vi "Dual_DM_Control_Main_V5.vi"() -> ()   [LabVIEW 2014]
uses:
  Controls/MirrorModes.ctl
  Controls/Standard Action.ctl
  <vilib>/Analysis/baseanly.llb/Mean (DBL).vi
  <vilib>/Utility/file.llb/Write To Spreadsheet File (DBL).vi
  <vilib>/Utility/file.llb/Read From Spreadsheet File (DBL).vi
  <vilib>/Analysis/NI_AALBase.lvlib
panel:
  in  "Control Mode":T1(radio)
  in  "Active Mirror":enum32{"Mirror 1", "Mirror 2"}(radio)
  in  "Clear Modes":bool
  in  "Mirror Modes":T2
  in  "Load Modes":bool
  in  "Save Modes":bool
  in  "Scan Modes":bool
  in  "Load Flat":bool
  in  "Apply Zero":bool
  in  "Load V Map":bool
  in  "Save V Map":bool
  in  "Apply Flat":bool
  in  "Center Bias":bool
  in  "Exit":bool
  out "Pixel Map (-1 to 1)":dbl[][](graph)
  # "Mode"
  # "Amount (nm)"
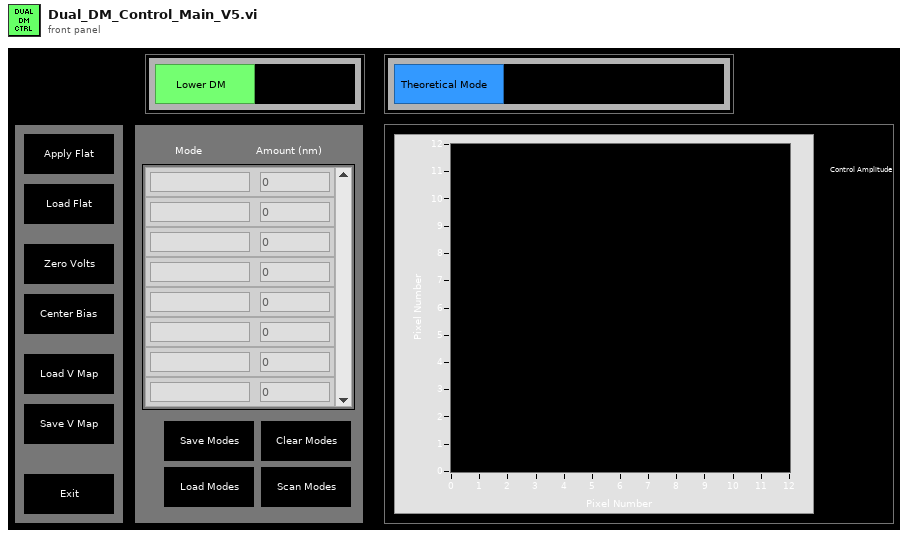
[diagram p1: front panel]
types:
  T1 = enum32{"Theoretical Mode", "Practical Mode", "Poke"}
  T2 = typedef "MirrorModes.ctl" = cluster{"Mode":string, "Amplitude":dbl}[]
  T3 = typedef "Standard Action.ctl" = enum16{"Read", "Write"}
  T4 = typedef "MirrorModes_DUAL.ctl" = cluster{"Mode":string, "Amplitude":dbl}[][]
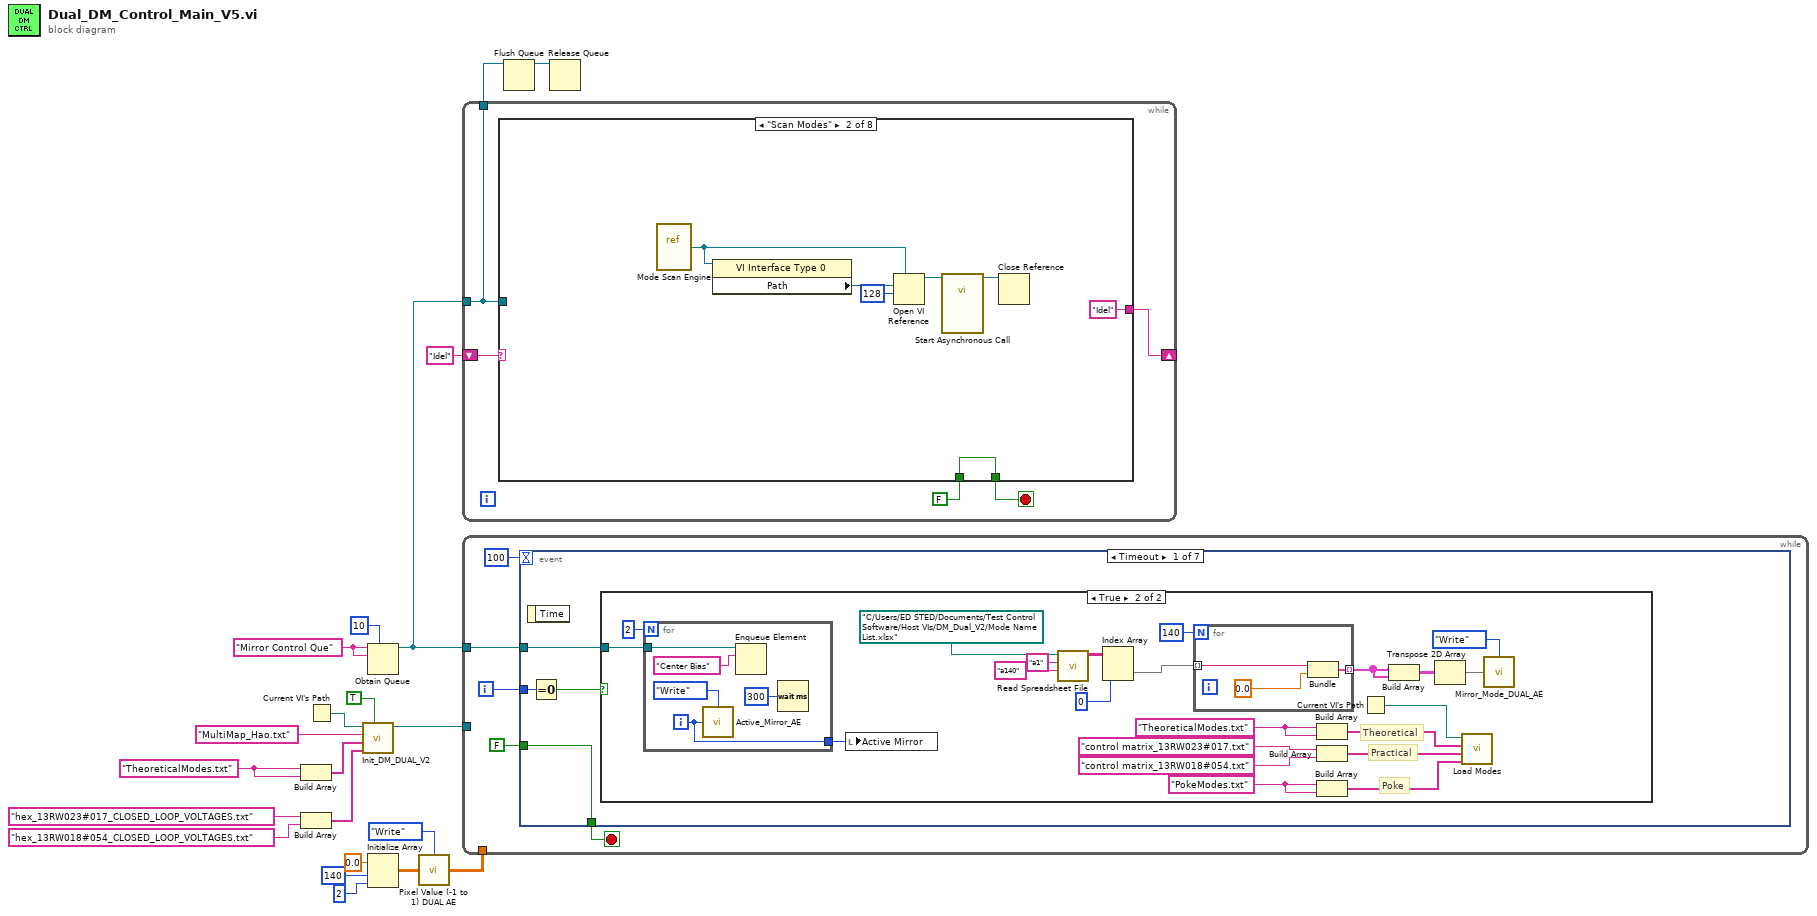
[diagram p0: block diagram]
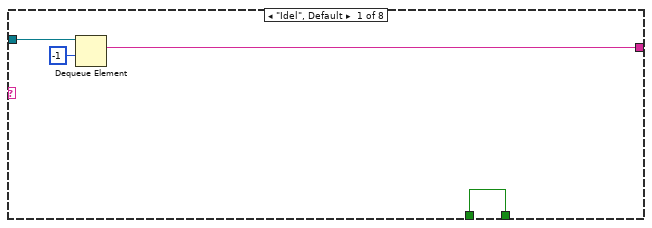
[diagram p2: hidden frame]
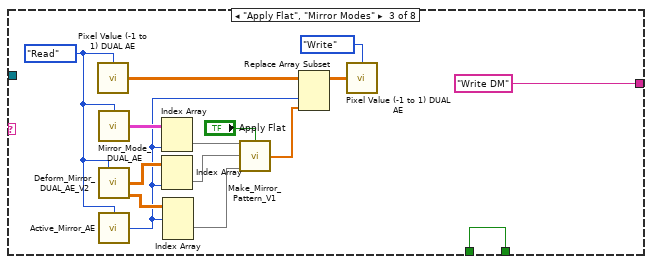
[diagram p3: hidden frame]
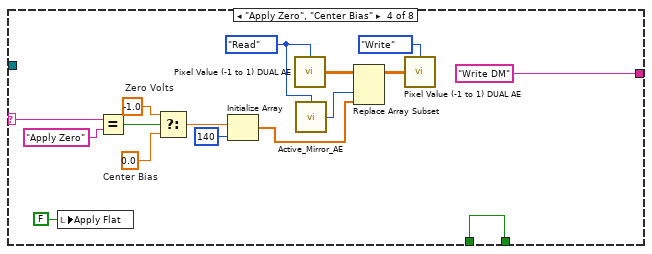
[diagram p4: hidden frame]
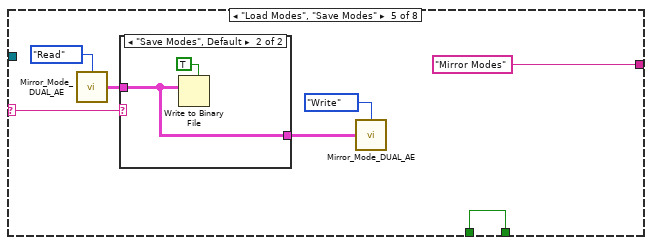
[diagram p5: hidden frame]
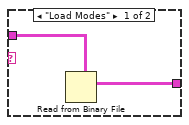
[diagram p6: hidden frame]
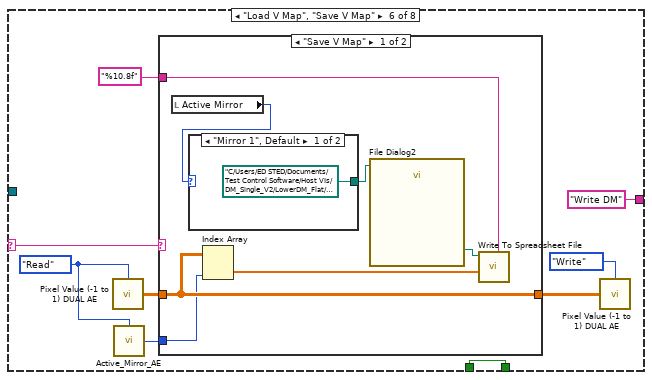
[diagram p7: hidden frame]
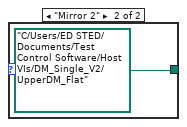
[diagram p8: hidden frame]
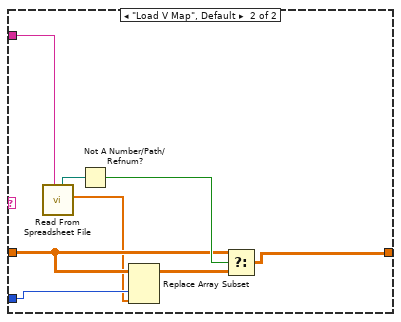
[diagram p9: hidden frame]
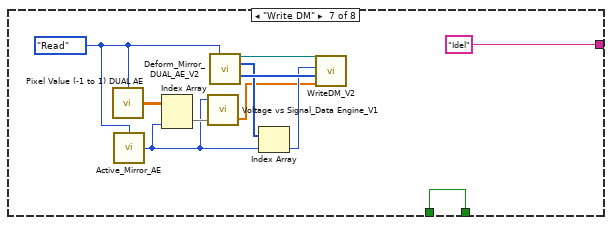
[diagram p10: hidden frame]
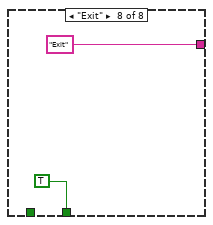
[diagram p11: hidden frame]
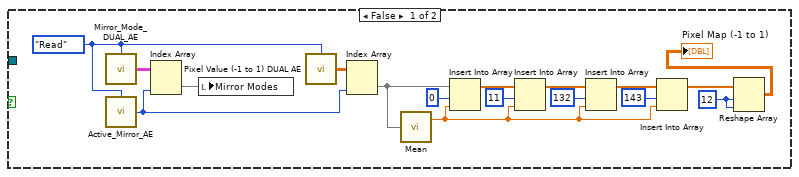
[diagram p12: hidden frame]
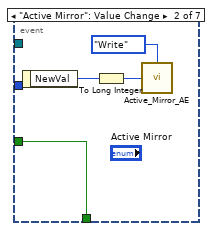
[diagram p13: hidden frame]
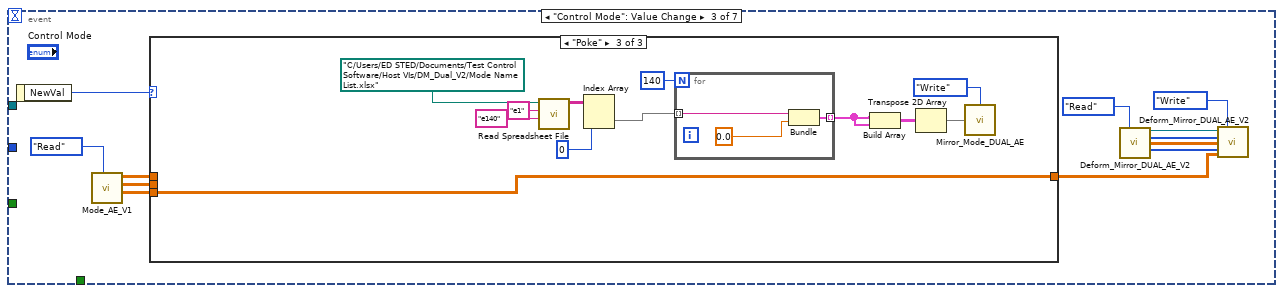
[diagram p14: hidden frame]
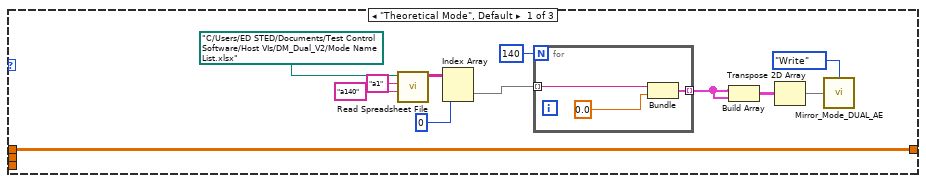
[diagram p15: hidden frame]
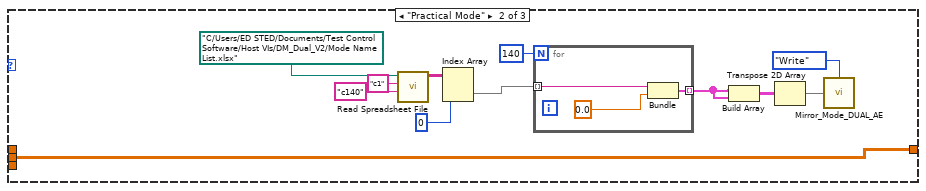
[diagram p16: hidden frame]
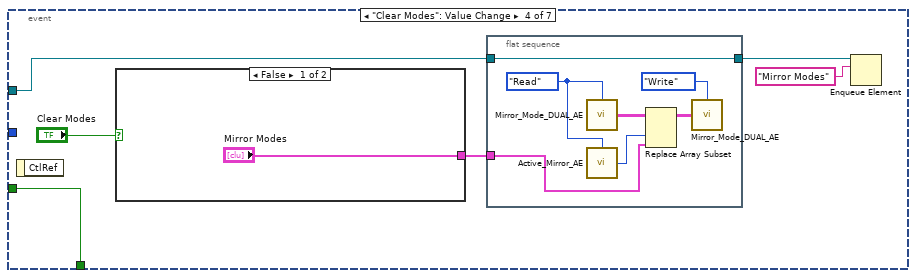
[diagram p17: hidden frame]
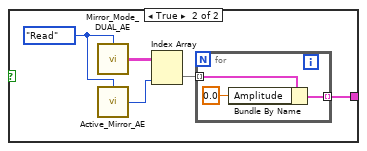
[diagram p18: hidden frame]
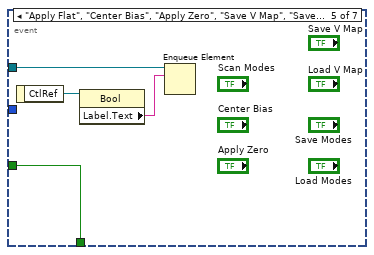
[diagram p19: hidden frame]
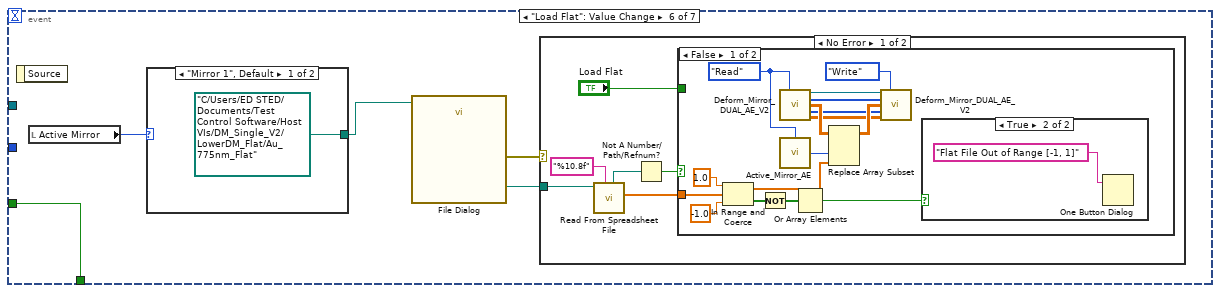
[diagram p20: hidden frame]
diagram:
  w1 = "TheoreticalModes.txt" ("name or relative path")
  w21 = "Mirror Control Que" ("name (unnamed)")
  n1 = Build Array(w1, w1) -> (w2:string[])
  n2 = Build Array("hex_13RW023#017_CLOSED_LOOP_VOLTAGES.txt" ("name or relative path"), "hex_13RW018#054_CLOSED_LOOP_VOLTAGES.txt" ("name or relative path")) -> (w11:string[])
  n3 = Current VI's Path() -> (path=w13:path)
  n4 = call "Init_DM_DUAL_V2.vi"("BM Flat"=TRUE, "BM Flat File"=w11, "Control Mode In"=w2, "DM Mapping File"="MultiMap_Hao.txt" ("name or relative path"), "Base File Path"=w13) -> ("reference out"=w19:refnum<k7>)  [unwired: 6 in]
  n5 = Obtain Queue(max queue size (-1, unlimited)=10, name (unnamed)=w21, element data type=w21) -> (queue out=w15:refnum<queue>)  [unwired: 2 in, 2 out]
  n6 = Initialize Array(0.0 ("element"), 140 ("dimension size"), 2 ("dimension size")) -> (w7:dbl[][])
  n7 = call "Pixel Value (-1 to 1) DUAL AE.vi"("Action"=Standard_Action."Write", "Pixel Value (-1 to 1)"=w7) -> ("Pixel Value (-1 to 1) Out"=w5:dbl[][])  [unwired: 13 in]
  n8 = while {
    tunnel: w15 -> [w22]
    shift-right: [w26] -> _
    shift-left: "Idel" ("name (unnamed)") -> [w25]
    tunnel: [w22] -> w18
    stop <- w24 stop-if-true
    n9 = case shown="\"Scan Modes\"" w25 {
      selector: w25 -> [_ _ _ w64 w71 w87 _ _]
      tunnel: w22 -> [w30 _ _ _ _ _ _ _]
      tunnel: [w28 "Idel" ("name (unnamed)") "Write DM" ("name (unnamed)") "Write DM" ("name (unnamed)") "Mirror Modes" ("name (unnamed)") "Write DM" ("name (unnamed)") "Idel" ("name (unnamed)") "Exit" ("name (unnamed)")] -> w26
      tunnel: [w27 w36 w51 w68 w75 w88 w116 TRUE] -> w24
      tunnel: FALSE -> [w27 w36 w51 w68 w75 w88 w116 _]
      frame "Idel", Default {
        n10 = Dequeue Element(queue=w30, timeout in ms (-1)=-1) -> (element=w28:string)  [unwired: 1 in, 3 out]
      }
      frame "Scan Modes" {
        n11 = vi-ref "Mode Scan Engine.vi"() -> (w31:refnum<vi>)
        n12 = property class="VI Interface Type 0"(reference=w31) -> ("Path"=w32:path)  [unwired: 1 in, 2 out]
        n13 = Open VI Reference(type specifier VI Refnum (for type only)=w31, vi path=w32, options=128) -> (vi reference=w34:refnum<vi>)  [unwired: 3 in, 1 out]
        n14 = call-by-ref "Start Asynchronous Call"(reference=w34) -> (reference out=w35:refnum<vi>)  [unwired: 3 in, 1 out]
        n15 = Close Reference(reference=w35) -> ()  [unwired: 1 in, 1 out]
      }
      frame "Apply Flat", "Mirror Modes" {
        w47 = Standard_Action."Read" ("Action")
        n16 = call "Pixel Value (-1 to 1) DUAL AE.vi"("Action"=w47) -> ("Pixel Value (-1 to 1) Out"=w48:dbl[][])  [unwired: 14 in]
        n17 = call "Mirror_Mode_DUAL_AE.vi"("Action"=w47) -> ("Mirror Modes Out"=w44:T4)  [unwired: 14 in]
        n18 = call "Deform_Mirror_DUAL_AE_V2.vi"("Action"=w47) -> ("Flat Files Out"=w42:dbl[][], "Mode Matrix Out"=w40:dbl[][][])  [unwired: 10 in, 3 out]
        n19 = call "Active_Mirror_AE.vi"("Action"=w47) -> ("Active Mirror"=w38:i32)  [unwired: 14 in]
        n20 = Index Array(array=w44, index (col)=w38) -> (element=w45:cluster{"Mode":string, "Amplitude":dbl}[])  [unwired: 1 in]
        n21 = Index Array(array=w42, index (col)=w38) -> (element=w43:dbl[])  [unwired: 1 in]
        n22 = Index Array(array=w40, index (dim 0)=w38) -> (element=w39:dbl[][])  [unwired: 2 in]
        n23 = call "Make_Mirror_Pattern_V1.vi"("Mirror Modes In"=w45, "Flat On?"="Apply Flat", "Flat File In"=w43, "Mirror Modes Array"=w39) -> ("Pixel Value U (-1 to 1)"=w49:dbl[])  [unwired: 11 in]
        n24 = Replace Array Subset(array=w48, new element=w49, index (col)=w38) -> (w50:dbl[][])  [unwired: 1 in]
        n25 = call "Pixel Value (-1 to 1) DUAL AE.vi"("Action"=Standard_Action."Write", "Pixel Value (-1 to 1)"=w50) -> ()  [unwired: 13 in, 1 out]
      }
      frame "Apply Zero", "Center Bias" {
        w57 = Standard_Action."Read" ("Action")
        w60 = -1.0  # Zero Volts
        w62 = 0.0  # Center Bias
        n26 = local write "Apply Flat"(FALSE ("Apply Flat")) -> ()
        n27 = Equal?(x=w64, y="Apply Zero") -> (x = y?=w63:bool)
        n28 = Select(t=w60, s=w63, f=w62) -> (s? t:f=w61:dbl)
        n29 = Initialize Array(w61, 140 ("dimension size")) -> (w54:dbl[])
        n30 = call "Pixel Value (-1 to 1) DUAL AE.vi"("Action"=w57) -> ("Pixel Value (-1 to 1) Out"=w55:dbl[][])  [unwired: 14 in]
        n31 = call "Active_Mirror_AE.vi"("Action"=w57) -> ("Active Mirror"=w56:i32)  [unwired: 14 in]
        n32 = Replace Array Subset(array=w55, new element=w54, index (col)=w56) -> (w58:dbl[][])  [unwired: 1 in]
        n33 = call "Pixel Value (-1 to 1) DUAL AE.vi"("Action"=Standard_Action."Write", "Pixel Value (-1 to 1)"=w58) -> ()  [unwired: 13 in, 1 out]
      }
      frame "Load Modes", "Save Modes" {
        n34 = call "Mirror_Mode_DUAL_AE.vi"("Action"=Standard_Action."Read") -> ("Mirror Modes Out"=w70:T4)  [unwired: 14 in]
        n35 = case shown="\"Save Modes\", Default" w71 {
          tunnel: w70 -> [w77 w78]
          tunnel: [w76 w78] -> w69
          frame "Load Modes" {
            n36 = Read from Binary File(5:w77) -> (2:w76:T4)  [unwired: 5 in, 3 out]
          }
          frame "Save Modes", Default {
            n37 = Write to Binary File(data=w78, 5:TRUE ("prepend array or string size? (T)")) -> ()  [unwired: 4 in, 3 out]
          }
        }
        n38 = call "Mirror_Mode_DUAL_AE.vi"("Action"=Standard_Action."Write", "Mirror Modes In"=w69) -> ()  [unwired: 13 in, 1 out]
      }
      frame "Load V Map", "Save V Map" {
        w81 = Standard_Action."Read" ("Action")
        n39 = call "Pixel Value (-1 to 1) DUAL AE.vi"("Action"=w81) -> ("Pixel Value (-1 to 1) Out"=w85:dbl[][])  [unwired: 14 in]
        n40 = call "Active_Mirror_AE.vi"("Action"=w81) -> ("Active Mirror"=w80:i32)  [unwired: 14 in]
        n41 = case shown="\"Save V Map\"" w87 {
          tunnel: w85 -> [w94 w101]
          tunnel: "%10.8f" -> [w95 w105]
          tunnel: [w94 w102] -> w82
          tunnel: w80 -> [w92 w100]
          frame "Save V Map" {
            n42 = local read "Active Mirror"() -> (w90:enum32{"Mirror 1", "Mirror 2"})
            n43 = case shown="\"Mirror 1\", Default" w90 {
              tunnel: [path "C:/Users/ED STED/Documents/Test Control Software/Host VIs/DM_Single_V2/LowerDM_Flat/Au_775nm_Flat" path "C:/Users/ED STED/Documents/Test Control Software/Host VIs/DM_Single_V2/UpperDM_Flat"] -> w89
              frame "Mirror 1", Default {
              }
              frame "Mirror 2" {
              }
            }
            n44 = Index Array(array=w94, index (col)=w92) -> (element=w93:dbl[])  [unwired: 1 in]
            n45 = call "File Dialog2"("start path"=w89) -> ("selected path"=w91:path)  [unwired: 11 in, 3 out]
            n46 = call-poly <vilib>:"Write To Spreadsheet File.vi"("format (%.3f)"=w95, "1D data"=w93, "file path (dialog if empty)"=w91) -> ()  [unwired: 5 in, 1 out]
          }
          frame "Load V Map", Default {
            n47 = call-poly <vilib>:"Read From Spreadsheet File.vi"("format (%.3f)"=w105) -> ("first row"=w99:dbl[], "new file path (Not A Path if cancelled)"=w104:path)  [unwired: 6 in, 3 out]
            n48 = Not A Number/Path/Refnum?(number/path/refnum=w104) -> (NaN/Path/Refnum?=w103:bool)
            n49 = Replace Array Subset(array=w101, new element=w99, index (col)=w100) -> (w98:dbl[][])  [unwired: 1 in]
            n50 = Select(t=w101, s=w103, f=w98) -> (s? t:f=w102:dbl[][])
          }
        }
        n51 = call "Pixel Value (-1 to 1) DUAL AE.vi"("Action"=Standard_Action."Write", "Pixel Value (-1 to 1)"=w82) -> ()  [unwired: 13 in, 1 out]
      }
      frame "Write DM" {
        w111 = Standard_Action."Read" ("Action")
        n52 = call "Pixel Value (-1 to 1) DUAL AE.vi"("Action"=w111) -> ("Pixel Value (-1 to 1) Out"=w112:dbl[][])  [unwired: 14 in]
        n53 = call "Active_Mirror_AE.vi"("Action"=w111) -> ("Active Mirror"=w106:i32)  [unwired: 14 in]
        n54 = Index Array(array=w112, index (col)=w106) -> (element=w107:dbl[])  [unwired: 1 in]
        n55 = call "Voltage vs Signal_Data Engine_V1.vi"("Control Signal In (-1~1)"=w107, "DM #"=w106) -> ("Voltage Out (0~Max. Vol.)"=w108:dbl[])  [unwired: 1 in, 1 out]
        n56 = call "Deform_Mirror_DUAL_AE_V2.vi"("Action"=w111) -> ("Refnum Out"=w114:refnum<k7>, "IDs Out"=w110:i32[], "Multi Map Data Out"=w113:i32[])  [unwired: 10 in, 2 out]
        n57 = Index Array(array=w110, index=w106) -> (element=w109:i32)
        n58 = call "WriteDM_V2.vi"("reference in"=w114, "nDevId"=w109, "MultiDM  Mapping"=w113, "Voltage Array in"=w108) -> ()  [unwired: 2 in, 2 out]
      }
      frame "Exit" {
      }
    }
  }
  n59 = while {
    tunnel: w15 -> [w119]
    tunnel: w19 -> [_]
    tunnel: w5 -> [_]
    i -> [w120]
    stop <- w123 stop-if-true
    n60 = event shown="[0] Timeout" {
      selector: _ -> [_ _ _ _ _ _ _]
      dyn-events: _ -> [_ _ _ _ _ _ _]
      timeout: 100 -> [_ _ _ _ _ _ _]
      tunnel: [w127 w178 _ w241 w261 w266 w303] -> w123
      tunnel: FALSE -> [w127 w178 _ w241 w261 w266 _]
      tunnel: w120 -> [w126 _ _ _ _ _ _]
      tunnel: w119 -> [w124 _ _ w240 w260 _ w301]
      event Timeout {
        n61 = event-data() -> ()  [unwired: 1 in, 1 out]
        n62 = Equal To 0?(x=w126) -> (x = 0?=w125:bool)
        n63 = case shown="True" w125 {
          tunnel: w124 -> [_ w166]
          frame False {
            w140 = 12 ("dimension size")
            w141 = Standard_Action."Read" ("Action")
            n64 = call "Mirror_Mode_DUAL_AE.vi"("Action"=w141) -> ("Mirror Modes Out"=w128:T4)  [unwired: 14 in]
            n65 = call "Active_Mirror_AE.vi"("Action"=w141) -> ("Active Mirror"=w143:i32)  [unwired: 14 in]
            n66 = Index Array(array=w128, index (col)=w143) -> (element=w129:cluster{"Mode":string, "Amplitude":dbl}[])  [unwired: 1 in]
            n67 = local write "Mirror Modes"(w129) -> ()
            n68 = call "Pixel Value (-1 to 1) DUAL AE.vi"("Action"=w141) -> ("Pixel Value (-1 to 1) Out"=w142:dbl[][])  [unwired: 14 in]
            n69 = Index Array(array=w142, index (col)=w143) -> (element=w144:dbl[])  [unwired: 1 in]
            n70 = call-poly <vilib>:"Mean.vi"("X"=w144) -> ("mean"=w138:dbl)  [unwired: 1 out]
            n71 = Insert Into Array(array=w144, index=0, new element=w138) -> (w133:dbl[])
            n72 = Insert Into Array(array=w133, index=11, new element=w138) -> (w135:dbl[])
            n73 = Insert Into Array(array=w135, index=132, new element=w138) -> (w137:dbl[])
            n74 = Insert Into Array(array=w137, index=143, new element=w138) -> (w130:dbl[])
            n75 = Reshape Array(w130, w140, w140) -> (→"Pixel Map (-1 to 1)":dbl[][])
          }
          frame True {
            w149 = "PokeModes.txt" ("name or relative path")
            w146 = "TheoreticalModes.txt" ("name or relative path")
            # "Poke"
            # "Practical"
            # "Theoretical"
            n76 = for {
              N: 2 -> [_]
              tunnel: w166 -> [w171]
              tunnel: [w167] -> w160
              i -> [w167]
              n77 = call "Active_Mirror_AE.vi"("Action"=Standard_Action."Write", "Active Mirror In"=w167) -> ()  [unwired: 13 in, 1 out]
              n78 = Enqueue Element(queue=w171, element="Center Bias") -> ()  [unwired: 2 in, 3 out]
              n79 = Wait (ms)(milliseconds to wait=u32 300) -> ()  [unwired: 1 out]
            }
            n80 = local write "Active Mirror"(w160) -> ()
            n81 = call "Read Spreadsheet File.vi"("End cell"="a140", "Start Cell"="a1", "path"=path "C:/Users/ED STED/Documents/Test Control Software/Host VIs/DM_Dual_V2/Mode Name List.xlsx") -> ("Array"=w155:string[][])  [unwired: 7 in, 1 out]
            n82 = Index Array(array=w155, index (col)=0 ("disabled index (col)")) -> (element=w153:string[])  [unwired: 1 in]
            n83 = for {
              N: 140 -> [_]
              tunnel: [w173] -> w163 mode=indexing
              tunnel: w153 -> [w172] mode=indexing
              n84 = Bundle(w172, 0.0) -> (w173:cluster{string, dbl})  [unwired: 1 in]
            }
            n85 = Build Array(w146, w146) -> (w151:string[])
            n86 = Build Array("control matrix_13RW023#017.txt" ("name or relative path"), "control matrix_13RW018#054.txt" ("name or relative path")) -> (w150:string[])
            n87 = Build Array(w149, w149) -> (w148:string[])
            n88 = Current VI's Path() -> (path=w152:path)
            n89 = Build Array(w163, w163) -> (w161:cluster{string, dbl}[][])
            n90 = Transpose 2D Array(2D array=w161) -> (transposed array=w156:cluster{string, dbl}[][])
            n91 = call "Load Modes.vi"("Poke Path"=w148, "Practical Mode Path"=w150, "Theoretical Mode Path"=w151, "Base File Path"=w152) -> ()  [unwired: 2 in]
            n92 = call "Mirror_Mode_DUAL_AE.vi"("Action"=Standard_Action."Write", "Mirror Modes In"=w156) -> ()  [unwired: 13 in, 1 out]
          }
        }
      }
      event "Active Mirror": Value Change {
        n93 = event-data() -> ("NewVal"=w177:enum32{"Mirror 1", "Mirror 2"})  [unwired: 1 in]
        n94 = To Long Integer(number=w177) -> (32bit integer=w176:i32)
        n95 = call "Active_Mirror_AE.vi"("Action"=Standard_Action."Write", "Active Mirror In"=w176) -> ()  [unwired: 13 in, 1 out]
      }
      event "Control Mode": Value Change {
        n96 = event-data() -> ("NewVal"=w190:T1)  [unwired: 1 in]
        n97 = call "Mode_AE_V1.vi"("Action"=Standard_Action."Read") -> ("Poke Mode Out"=w185:dbl[][][], "Practical Mode Out"=w186:dbl[][][], "Theoretical Mode Out"=w187:dbl[][][])  [unwired: 7 in]
        n98 = case shown="\"Poke\"" w190 {
          tunnel: w187 -> [w202 _ _]
          tunnel: w186 -> [_ w217 _]
          tunnel: w185 -> [_ _ w221]
          tunnel: [w202 w217 w221] -> w184
          frame "Theoretical Mode", Default {
            n99 = call "Read Spreadsheet File.vi"("End cell"="a140", "Start Cell"="a1", "path"=path "C:/Users/ED STED/Documents/Test Control Software/Host VIs/DM_Dual_V2/Mode Name List.xlsx") -> ("Array"=w193:string[][])  [unwired: 7 in, 1 out]
            n100 = Index Array(array=w193, index (col)=0 ("disabled index (col)")) -> (element=w191:string[])  [unwired: 1 in]
            n101 = for {
              N: 140 -> [_]
              tunnel: [w204] -> w199 mode=indexing
              tunnel: w191 -> [w203] mode=indexing
              n102 = Bundle(w203, 0.0) -> (w204:cluster{string, dbl})  [unwired: 1 in]
            }
            n103 = Build Array(w199, w199) -> (w198:cluster{string, dbl}[][])
            n104 = Transpose 2D Array(2D array=w198) -> (transposed array=w194:cluster{string, dbl}[][])
            n105 = call "Mirror_Mode_DUAL_AE.vi"("Action"=Standard_Action."Write", "Mirror Modes In"=w194) -> ()  [unwired: 13 in, 1 out]
          }
          frame "Practical Mode" {
            n106 = call "Read Spreadsheet File.vi"("End cell"="c140", "Start Cell"="c1", "path"=path "C:/Users/ED STED/Documents/Test Control Software/Host VIs/DM_Dual_V2/Mode Name List.xlsx") -> ("Array"=w208:string[][])  [unwired: 7 in, 1 out]
            n107 = Index Array(array=w208, index (col)=0 ("disabled index (col)")) -> (element=w206:string[])  [unwired: 1 in]
            n108 = for {
              N: 140 -> [_]
              tunnel: [w219] -> w214 mode=indexing
              tunnel: w206 -> [w218] mode=indexing
              n109 = Bundle(w218, 0.0) -> (w219:cluster{string, dbl})  [unwired: 1 in]
            }
            n110 = Build Array(w214, w214) -> (w213:cluster{string, dbl}[][])
            n111 = Transpose 2D Array(2D array=w213) -> (transposed array=w209:cluster{string, dbl}[][])
            n112 = call "Mirror_Mode_DUAL_AE.vi"("Action"=Standard_Action."Write", "Mirror Modes In"=w209) -> ()  [unwired: 13 in, 1 out]
          }
          frame "Poke" {
            n113 = call "Read Spreadsheet File.vi"("End cell"="e140", "Start Cell"="e1", "path"=path "C:/Users/ED STED/Documents/Test Control Software/Host VIs/DM_Dual_V2/Mode Name List.xlsx") -> ("Array"=w224:string[][])  [unwired: 7 in, 1 out]
            n114 = Index Array(array=w224, index (col)=0 ("disabled index (col)")) -> (element=w222:string[])  [unwired: 1 in]
            n115 = for {
              N: 140 -> [_]
              tunnel: [w234] -> w230 mode=indexing
              tunnel: w222 -> [w233] mode=indexing
              n116 = Bundle(w233, 0.0) -> (w234:cluster{string, dbl})  [unwired: 1 in]
            }
            n117 = Build Array(w230, w230) -> (w229:cluster{string, dbl}[][])
            n118 = Transpose 2D Array(2D array=w229) -> (transposed array=w225:cluster{string, dbl}[][])
            n119 = call "Mirror_Mode_DUAL_AE.vi"("Action"=Standard_Action."Write", "Mirror Modes In"=w225) -> ()  [unwired: 13 in, 1 out]
          }
        }
        n120 = call "Deform_Mirror_DUAL_AE_V2.vi"("Action"=Standard_Action."Read") -> ("Refnum Out"=w183:refnum<k7>, "IDs Out"=w182:i32[], "Flat Files Out"=w181:dbl[][], "Multi Map Data Out"=w180:i32[])  [unwired: 10 in, 1 out]
        n121 = call "Deform_Mirror_DUAL_AE_V2.vi"("Refnum In"=w183, "Action"=Standard_Action."Write", "IDs In"=w182, "Flat Files In"=w181, "Multi Map Data In"=w180, "Mode Matrix In"=w184) -> ()  [unwired: 5 in, 5 out]
      }
      event "Clear Modes": Value Change {
        n122 = event-data() -> ()  [unwired: 1 in, 1 out]
        n123 = case shown="False" "Clear Modes" {
          tunnel: ["Mirror Modes" w243] -> w236
          frame False {
          }
          frame True {
            w246 = Standard_Action."Read" ("Action")
            n124 = call "Mirror_Mode_DUAL_AE.vi"("Action"=w246) -> ("Mirror Modes Out"=w245:T4)  [unwired: 14 in]
            n125 = call "Active_Mirror_AE.vi"("Action"=w246) -> ("Active Mirror"=w247:i32)  [unwired: 14 in]
            n126 = Index Array(array=w245, index (col)=w247) -> (element=w244:cluster{"Mode":string, "Amplitude":dbl}[])  [unwired: 1 in]
            n127 = for {
              tunnel: w244 -> [w250] mode=indexing
              tunnel: [w248] -> w243 mode=indexing
              n128 = Bundle By Name(cluster=w250, "Amplitude"=0.0) -> (w248:cluster{"Mode":string, "Amplitude":dbl})
            }
          }
        }
        n129 = flat-sequence {
          tunnel: w236 -> [w251]
          tunnel: w240 -> [w257]
          tunnel: [w257] -> w238
          frame #0 {
            w254 = Standard_Action."Read" ("Action")
            n130 = call "Mirror_Mode_DUAL_AE.vi"("Action"=w254) -> ("Mirror Modes Out"=w253:T4)  [unwired: 14 in]
            n131 = call "Active_Mirror_AE.vi"("Action"=w254) -> ("Active Mirror"=w255:i32)  [unwired: 14 in]
            n132 = Replace Array Subset(array=w253, new element=w251, index (col)=w255) -> (w256:T4)  [unwired: 1 in]
            n133 = call "Mirror_Mode_DUAL_AE.vi"("Action"=Standard_Action."Write", "Mirror Modes In"=w256) -> ()  [unwired: 13 in, 1 out]
          }
        }
        n134 = Enqueue Element(queue=w238, element="Mirror Modes") -> ()  [unwired: 2 in, 3 out]
      }
      event "Apply Flat", "Center Bias", "Apply Zero", "Save V Map", "Save Modes", "Load Modes", "Load V Map", "Scan Modes": Value Change {
        n135 = event-data() -> ("CtlRef"=w259:refnum<vi>)  [unwired: 1 in]
        n136 = property class="Bool"(reference=w259) -> ("Label.Text"=w258:string)  [unwired: 1 in, 2 out]
        n137 = Enqueue Element(queue=w260, element=w258) -> ()  [unwired: 2 in, 3 out]
      }
      event "Load Flat": Value Change {
        n138 = event-data() -> ()  [unwired: 1 in, 1 out]
        n139 = local read "Active Mirror"() -> (w264:enum32{"Mirror 1", "Mirror 2"})
        n140 = case shown="\"Mirror 1\", Default" w264 {
          tunnel: [path "C:/Users/ED STED/Documents/Test Control Software/Host VIs/DM_Single_V2/LowerDM_Flat/Au_775nm_Flat" path "C:/Users/ED STED/Documents/Test Control Software/Host VIs/DM_Single_V2/UpperDM_Flat"] -> w263
          frame "Mirror 1", Default {
          }
          frame "Mirror 2" {
          }
        }
        n141 = call "File Dialog"("start path"=w263) -> ("selected path"=w265:path, "error out"=w262:errorcluster)  [unwired: 11 in, 2 out]
        n142 = case shown="No Error" w262 {
          tunnel: w265 -> [w267 _]
          frame No Error {
            n143 = call-poly <vilib>:"Read From Spreadsheet File.vi"("format (%.3f)"="%10.8f", "file path (dialog if empty)"=w267) -> ("first row"=w269:dbl[], "new file path (Not A Path if cancelled)"=w271:path)  [unwired: 5 in, 3 out]
            n144 = Not A Number/Path/Refnum?(number/path/refnum=w271) -> (NaN/Path/Refnum?=w270:bool)
            n145 = case shown="False" w270 {
              tunnel: w269 -> [w288 _]
              tunnel: "Load Flat" -> [_ _]
              frame False {
                w279 = Standard_Action."Read" ("Action")
                n146 = In Range and Coerce(upper limit=1.0, x=w288, lower limit=-1.0) -> (coerced(x)=w273:dbl[], In Range?=w285:bool[])
                n147 = Not(x=w285) -> (.not. x?=w284:bool[])
                n148 = call "Deform_Mirror_DUAL_AE_V2.vi"("Action"=w279) -> ("Refnum Out"=w274:refnum<k7>, "IDs Out"=w275:i32[], "Flat Files Out"=w280:dbl[][], "Multi Map Data Out"=w276:i32[], "Mode Matrix Out"=w277:dbl[][][])  [unwired: 10 in]
                n149 = call "Active_Mirror_AE.vi"("Action"=w279) -> ("Active Mirror"=w282:i32)  [unwired: 14 in]
                n150 = Or Array Elements(Boolean array=w284) -> (logical OR=w283:bool)
                n151 = Replace Array Subset(array=w280, new element=w273, index (col)=w282) -> (w281:dbl[][])  [unwired: 1 in]
                n152 = call "Deform_Mirror_DUAL_AE_V2.vi"("Refnum In"=w274, "Action"=Standard_Action."Write", "IDs In"=w275, "Flat Files In"=w281, "Multi Map Data In"=w276, "Mode Matrix In"=w277) -> ()  [unwired: 5 in, 5 out]
                n153 = case shown="True" w283 {
                  frame False {
                  }
                  frame True {
                    n154 = One Button Dialog(message="Flat File Out of Range [-1, 1]") -> ()  [unwired: 1 in, 1 out]
                  }
                }
              }
              frame True {
              }
            }
          }
          frame Error {
          }
        }
      }
      event "Exit": Value Change {
        n155 = event-data() -> ("NewVal"=w303:bool)  [unwired: 1 in]
        n156 = for {
          N: 2 -> [_]
          tunnel: w301 -> [w309]
          tunnel: [w304] -> w292
          i -> [w305]
          n157 = call "Active_Mirror_AE.vi"("Action"=Standard_Action."Write", "Active Mirror In"=w305) -> ()  [unwired: 13 in, 1 out]
          n158 = Enqueue Element(queue=w309, element="Apply Zero") -> (queue out=w304:refnum<queue>)  [unwired: 2 in, 2 out]
          n159 = Wait (ms)(milliseconds to wait=u32 300) -> ()  [unwired: 1 out]
        }
        n160 = Enqueue Element(queue=w292, element="Exit") -> (error out=w296:errorcluster)  [unwired: 2 in, 2 out]
        n161 = call "Deform_Mirror_DUAL_AE_V2.vi"("Action"=Standard_Action."Read") -> ("Refnum Out"=w299:refnum<k7>, "IDs Out"=w294:i32[])  [unwired: 10 in, 3 out]
        n162 = call "ConfigDM.vi"("High Voltage"=FALSE, "error in (no error)"=w296, "Dev IDs"=w294, "Automation Refnum in"=w299) -> ("error out"=w295:errorcluster, "Automation Refnum out"=w298:refnum<k7>)  [unwired: 6 in]
        n163 = Close Reference(reference=w298, error in (no error)=w295) -> ()  [unwired: 1 out]
      }
    }
  }
  n164 = Flush Queue(queue=w18) -> (queue out=w17:refnum<queue>)  [unwired: 1 in, 2 out]
  n165 = Release Queue(queue=w17) -> ()  [unwired: 2 in, 3 out]
